vi "Read Address Pointer - 12bit with overflow.vi"(9 "INC?":bool, 10 "Read Pointer Offset":u16) -> (1 "Read Pointer":u32, 3 "Write Pointer":u32)   [LabVIEW 2014]
panel:
  # "Copyright 2014 Vidrio Technologies\nScanImage 5 software is licensed under the Apache License, Version 2.0 (the \"License\"); you may not use any files contained\nwithin the ScanImage 5 release except in compliance with the License. You may obtain a copy of the License at\n http://www.apache.org/licenses/LICENSE-2.0\nUnless required by applicable law or agreed to in writing, software distributed under the License is distributed on an\n\"AS IS\" BASIS, WITHOUT WARRANTIES OR CONDITIONS OF ANY KIND, either express or implied. See the License for the\n specific language governing permissions and limitations under the License."
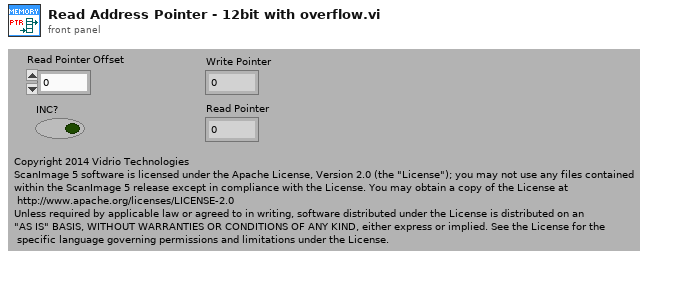
[diagram p1: front panel]
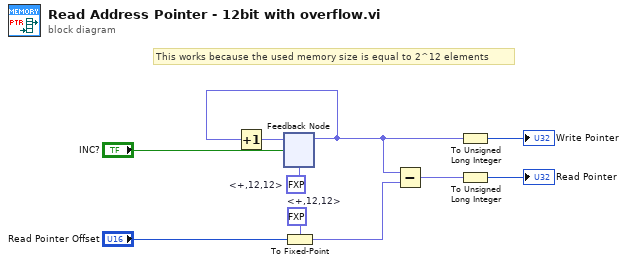
[diagram p0: block diagram]
diagram:
  w4 = fxp<+,12,12> 0.0  # <+,12,12>
  w7 = fxp<+,12,12> 0.0  # <+,12,12>
  # "This works because the used memory size is equal to 2^12 elements"
  n1 = feedback #1(w7) -> (w1:fxp<+,12,12>)
  n2 = Increment(x=w1) -> (x+1=w8:fxp<+,12,12>)
  n3 = feedback-in #1(w8, "INC?") -> ()
  n4 = To Fixed-Point(fixed-point type=w4, number="Read Pointer Offset") -> (fixed-point=w9:fxp<+,12,12>)
  n5 = Subtract(x=w1, y=w9) -> (x-y=w5:fxp<+,12,12>)
  n6 = To Unsigned Long Integer(number=w1) -> (unsigned 32bit integer=→"Write Pointer":u32)
  n7 = To Unsigned Long Integer(number=w5) -> (unsigned 32bit integer=→"Read Pointer":u32)
